vi "Draw Star.vi"(6 "Draw Para":T1={"fill?(F)"=TRUE, "color(black)"=0, "pen"={"Width"=1, "Style"=enum."Solid"}}, 7 "Angle":dbl=10.0, 8 "错误输入":errorcluster, 9 "Radius":i16=10, 10 "Center":T2, 11 "Pic in":picture) -> (0 "错误输出":errorcluster, 3 "Pic out":picture)   [LabVIEW 2011, in "Basic Shape.lvlib"]
uses:
  Basic Shape.lvlib
  Point Custom Control.ctl
  Draw Para Custom Control.ctl
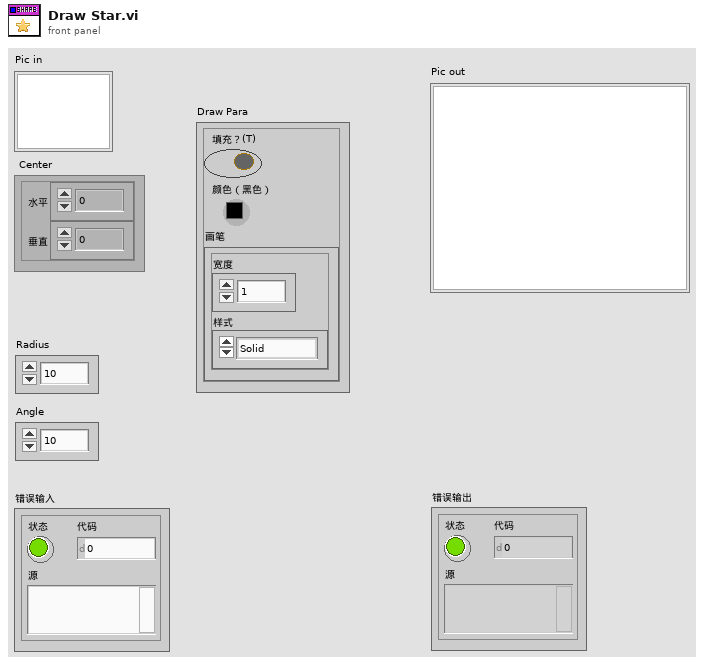
[diagram p1: front panel]
types:
  T1 = typedef "Basic Shape.lvlib/Draw Para Custom Control.ctl" = cluster{"fill?(F)":bool, "color(black)":u32, "pen":cluster{"Width":u16, "Style":enum32{"Solid", "Dash", "Dot", "DashDot", "DashDotDot"}}}
  T2 = typedef "Basic Shape.lvlib/Point Custom Control.ctl" = cluster{"horizontal":i16, "vertical":i16}
  T3 = cluster{"Radius":i16, "Divisions":i16, "Closed":bool}
  T4 = cluster{"Width":u16, "Style":enum32{"Solid", "Dash", "Dot", "DashDot", "DashDotDot"}}
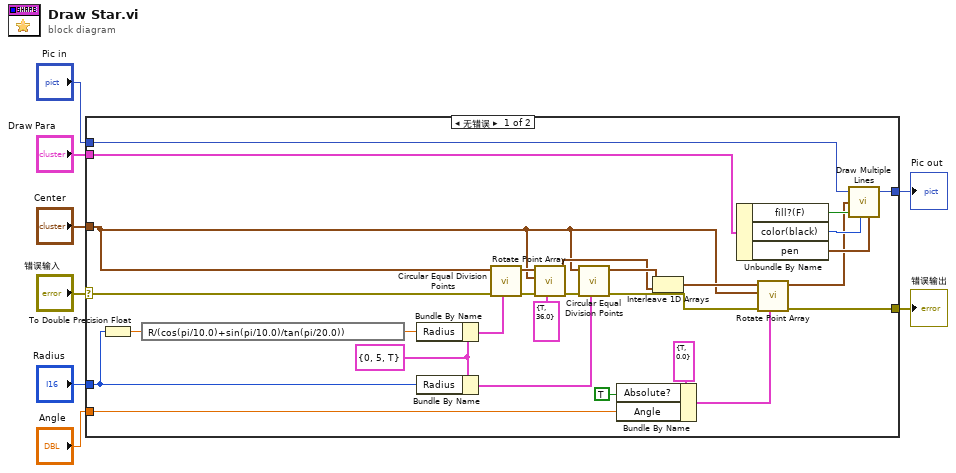
[diagram p0: block diagram]
diagram:
  n1 = case shown="无错误" "错误输入" {
    selector: "错误输入" -> [w21 w38]
    tunnel: [w16 w38] -> w7
    tunnel: "Center" -> [w15 _]
    tunnel: "Pic in" -> [w27 w37]
    tunnel: [w24 w37] -> w4
    tunnel: "Draw Para" -> [w36 _]
    tunnel: "Radius" -> [w35 _]
    tunnel: "Angle" -> [w12 _]
    frame No Error {
      w23 = T3 {"Radius"=0, "Divisions"=5, "Closed"=TRUE} ("Para")
      n2 = To Double Precision Float(number=w35) -> (double precision float=w28:dbl)
      n3 = expression code="R/(cos(pi/10.0)+sin(pi/10.0)/tan(pi/20.0))"(w28) -> (w9:dbl)
      n4 = Bundle By Name(cluster=w23, "Radius"=w9) -> (w34:T3)
      n5 = Bundle By Name(cluster=w23, "Radius"=w35) -> (w22:T3)
      n6 = call "Circular Equal Division Points.vi"("Para"=w34, "错误输入"=w21, "Center"=w15) -> ("错误输出"=w31:errorcluster, "Absolute Point Array"=w30:T2[])  [unwired: 6 in, 1 out]
      n7 = call "Rotate Point Array.vi"("Para"=cluster{"Absolute?":bool, "Angle":dbl} {"Absolute?"=TRUE, "Angle"=36.0}, "错误输入"=w31, "Center"=w15, "Point Array"=w30) -> ("错误输出"=w20:errorcluster, "Rotated Absolute Point Array"=w25:T2[])  [unwired: 5 in, 1 out]
      n8 = call "Circular Equal Division Points.vi"("Para"=w22, "错误输入"=w20, "Center"=w15) -> ("错误输出"=w17:errorcluster, "Absolute Point Array"=w26:T2[])  [unwired: 6 in, 1 out]
      n9 = Bundle By Name(cluster=cluster{"Absolute?":bool, "Angle":dbl} {"Absolute?"=TRUE, "Angle"=0.0} ("Para"), "Absolute?"=TRUE, "Angle"=w12) -> (w10:cluster{"Absolute?":bool, "Angle":dbl})
      n10 = Interleave 1D Arrays(w26, w25) -> (w18:T2[])
      n11 = Unbundle By Name(w36) -> ("fill?(F)"=w19:bool, "color(black)"=w33:u32, "pen"=w32:T4)
      n12 = call "Rotate Point Array.vi"("Para"=w10, "错误输入"=w17, "Center"=w15, "Point Array"=w18) -> ("错误输出"=w16:errorcluster, "Rotated Absolute Point Array"=w11:T2[])  [unwired: 5 in, 1 out]
      n13 = call <vilib>:"Draw Multiple Lines.vi"("picture"=w27, "line endpoints"=w11, "fill?(F)"=w19, "color(black)"=w33, "pen"=w32) -> ("new picture"=w24:picture)  [unwired: 4 in]
    }
    frame Error {
    }
  }
  "Pic out" <- w4
  "错误输出" <- w7
